vi "Write Build Machine Feed Folder path.vi"(8 "error in (no error)":errorcluster, 10 "Build Machine Feed Folder path":path, 11 "CommitNIPKG_LV in":refnum<class "CommitNIPKG_LV.lvclass">) -> (0 "error out":errorcluster, 3 "CommitNIPKG_LV out":refnum<class "CommitNIPKG_LV.lvclass">)   [LabVIEW 2017, in "CL_G3_VIComponentBuilder.lvlib" / "CommitNIPKG_LV.lvclass"]
uses:
  CommitNIPKG_LV.lvclass
  CommitNIPKG_LV.lvclass/CommitNIPKG_LV.ctl
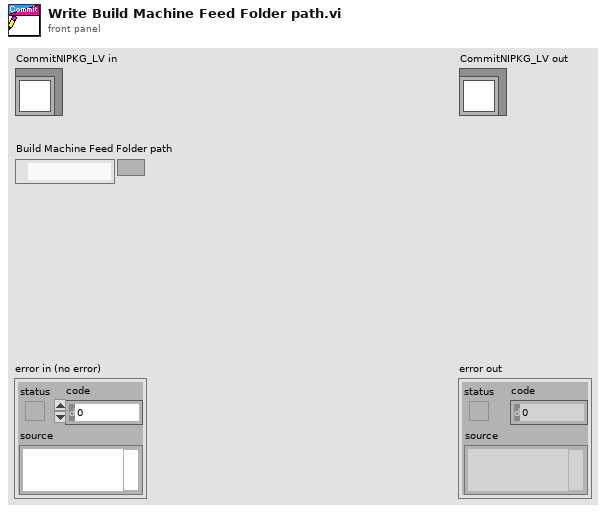
[diagram p1: front panel]
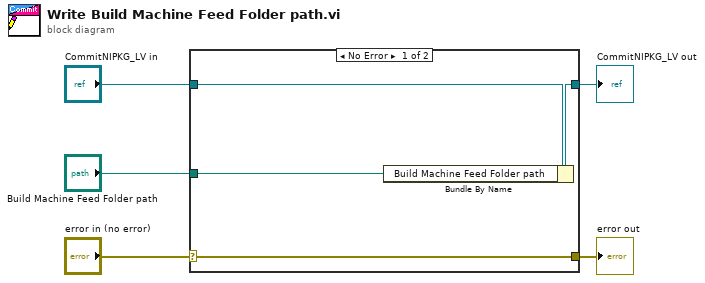
[diagram p0: block diagram]
diagram:
  n1 = case shown="No Error" "error in (no error)" {
    selector: "error in (no error)" -> [w9 w10]
    tunnel: [w9 w10] -> w4
    tunnel: [w7 w11] -> w2
    tunnel: "CommitNIPKG_LV in" -> [w8 w11]
    tunnel: "Build Machine Feed Folder path" -> [w6 _]
    frame No Error {
      n2 = Bundle By Name(cluster=w8, "Build Machine Feed Folder path"=w6) -> (w7:refnum<class "CommitNIPKG_LV.lvclass">)
    }
    frame Error {
    }
  }
  "error out" <- w4
  "CommitNIPKG_LV out" <- w2
